vi "Initialize.vi"(5 "TimeZoneInfoId":string, 6 "MeasureExecutionStatus":T2=enum."NOT_COMPLETED", 7 "MeasureTime":timestamp, 8 "error in":errorcluster, 9 "Type":T1, 10 "Name":string, 11 "Measure in":refnum<class "Measure.lvclass">) -> (0 "error out":errorcluster, 3 "Measure out":refnum<class "Measure.lvclass">)   [LabVIEW 2021, in "ProligentXMLGenerator.lvlib" / "Measure.lvclass"]
uses:
  Measure.lvclass
  Measure.lvclass/Measure.ctl
  Base/DateTime/DateTime.lvclass
  Base/ExecutionStatus/ExecutionStatus.lvclass
  Data.ctl
  Base/MeasureKind/MeasureKind.lvclass
  MeasureLimit/MeasureLimit.lvclass
  Base/NonEmptyString_20/NonEmptyString_20.lvclass
  Base/NonEmptyString_30/NonEmptyString_30.lvclass
  Base/NonNullableString_TruncateAt_255/NonNullableString_TruncateAt_255.lvclass
  Base/Guid/Guid.lvclass
  Model/CustomData/CustomData.lvclass
  Failure/FailureReference/FailureReference.lvclass
  Model/Characteristic/Characteristic.lvclass
  Base/UnsignedByte/UnsignedByte.lvclass
  Base/ExecutionStatus/Value.ctl
  Base/MeasureKind/Value.ctl
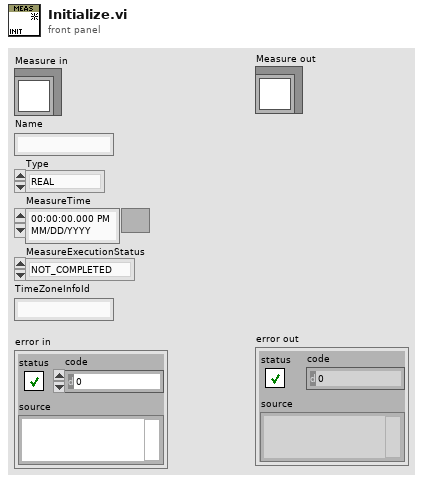
[diagram p1: front panel]
types:
  T1 = typedef "ProligentXMLGenerator.lvlib/MeasureKind.lvclass/Value.ctl" = enum16{"REAL", "BOOL", "INTEGER", "STRING", "DATETIME"}
  T2 = typedef "ProligentXMLGenerator.lvlib/ExecutionStatus.lvclass/Value.ctl" = enum16{"PASS", "FAIL", "NOT_COMPLETED", "ABORTED"}
  T3 = typedef "ProligentXMLGenerator.lvlib/Measure.lvclass/Data.ctl" = cluster{"Name":string, "Type":refnum<class "MeasureKind.lvclass">, "Precision":refnum<class "UnsignedByte.lvclass">, "Limit":refnum<class "MeasureLimit.lvclass">, "Characteristics":refnum<class "Characteristic.lvclass">[], "FailureReferences":refnum<class "FailureReference.lvclass">[], "CustomData":refnum<class "CustomData.lvclass">, "MeasureId":refnum<class "Guid.lvclass">, "MeasureTime":refnum<class "DateTime.lvclass">, "Comments":refnum<class "NonNullableString_TruncateAt_255.lvclass">, "Unit":refnum<class "NonEmptyString_30.lvclass">, "Symbol":refnum<class "NonEmptyString_20.lvclass">, "MeasureExecutionStatus":refnum<class "ExecutionStatus.lvclass">}
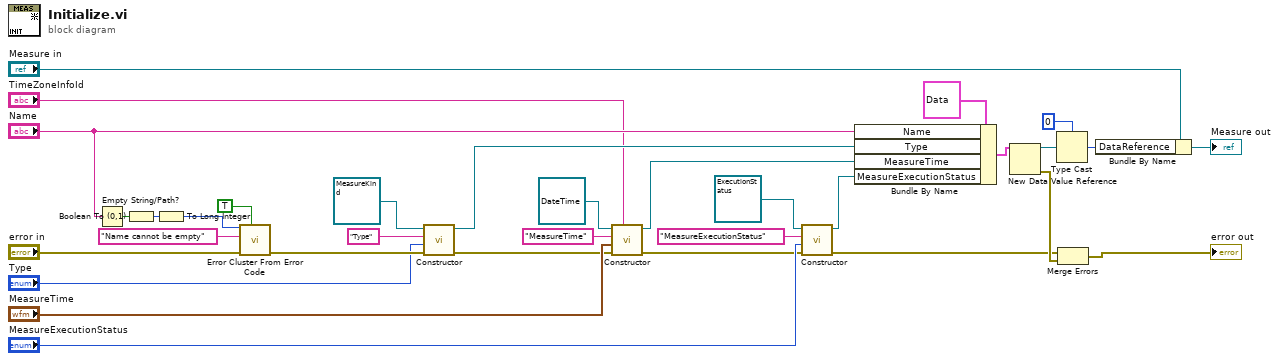
[diagram p0: block diagram]
diagram:
  n1 = Empty String/Path?(string/path="Name") -> (empty?=w20:bool)
  n2 = Boolean To (0,1)(Boolean=w20) -> (0, 1=w19:i16)
  n3 = To Long Integer(number=w19) -> (32bit integer=w18:i32)
  n4 = call <vilib>:"Error Cluster From Error Code.vi"("show call chain? (False)"=TRUE, "error in (no error)"="error in", "error message (\"\")"="Name cannot be empty" ("error message (\"\")"), "error code (0)"=w18) -> ("error out"=w9:errorcluster)  [unwired: 5 in]
  n5 = call-dynamic "Constructor.vi"("error in"=w9, "Value"="Type", "Name"="Type", "Measure in"=refnum<class "MeasureKind.lvclass"> refnum ("ProligentResultProcessor:MeasureKind")) -> ("error out"=w3:errorcluster, "Measure out"=w7:refnum<class "MeasureKind.lvclass">)  [unwired: 6 in]
  n6 = call-dynamic "Constructor.vi"("TimeZoneInfoId"="TimeZoneInfoId", "error in"=w3, "Value"="MeasureTime", "Name"="MeasureTime", "DateTime in"=refnum<class "DateTime.lvclass"> refnum) -> ("error out"=w2:errorcluster, "DateTime out"=w11:refnum<class "DateTime.lvclass">)  [unwired: 5 in]
  n7 = call-dynamic "Constructor.vi"("error in"=w2, "Value"="MeasureExecutionStatus", "Name"="MeasureExecutionStatus", "ExecutionStatus in"=refnum<class "ExecutionStatus.lvclass"> refnum ("ProligentResultProcessor:ExecutionStatus")) -> ("error out"=w12:errorcluster, "ExecutionStatus out"=w14:refnum<class "ExecutionStatus.lvclass">)  [unwired: 6 in]
  n8 = Bundle By Name(cluster=T3 {"Name"="", "Type"=refnum, "Precision"=refnum, "Limit"=refnum, "Characteristics"=[], "FailureReferences"=[], "CustomData"=refnum, "MeasureId"=refnum, "MeasureTime"=refnum, "Comments"=refnum, "Unit"=refnum, "Symbol"=refnum, "MeasureExecutionStatus"=refnum} ("Data"), "Name"="Name", "Type"=w7, "MeasureTime"=w11, "MeasureExecutionStatus"=w14) -> (w26:T3)
  n9 = New Data Value Reference(data value=w26) -> (data value reference=w25:refnum<data-value>, error out=w22:errorcluster)  [unwired: 1 in]
  n10 = Type Cast(type=u64 0, x=w25) -> (*(type *) &x=w23:u64)
  n11 = Merge Errors(w12, w22) -> (→"error out":errorcluster)
  n12 = Bundle By Name(cluster="Measure in", "DataReference"=w23) -> (→"Measure out":refnum<class "Measure.lvclass">)
